vi "Read Excel data.vi"() -> (0 "Number of rows":i32, 1 "Plot Group":dbl[][](array[numeric]), 2 "Voltage Offsets":dbl[][](array[numeric]), 3 "Chirp Durations":dbl[][](array[numeric]))   [LabVIEW 2017]
uses:
  <vilib>/Utility/file.llb/Read Delimited Spreadsheet (DBL).vi
panel:
  out "array w/o headers":dbl[][](array[numeric])
  out "all rows":dbl[][](array[numeric])
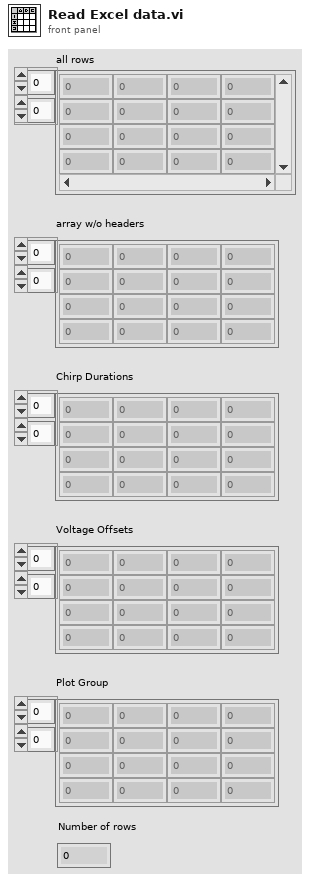
[diagram p1: front panel]
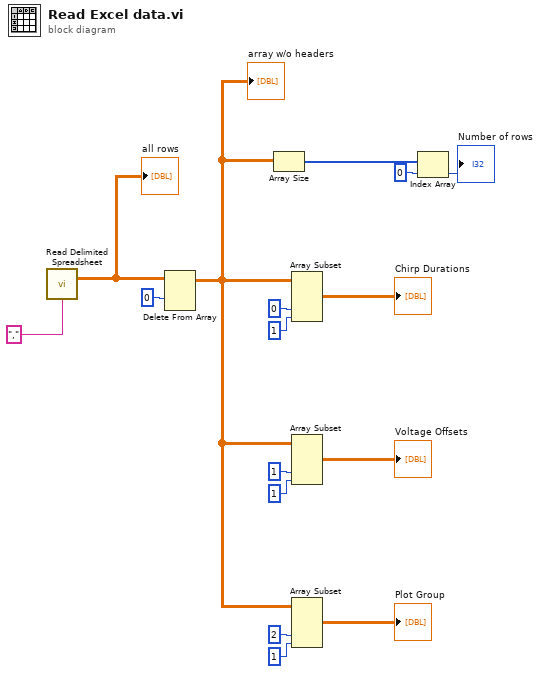
[diagram p0: block diagram]
diagram:
  n1 = call-poly <vilib>:"Read Delimited Spreadsheet.vi"("delimiter (\\t)"="," ("delimiter (\\t)")) -> ("all rows"=w16:dbl[][])  [unwired: 9 in, 5 out]
  "all rows" <- w16
  n2 = Delete From Array(array=w16, index (row)=0) -> (array with subset deleted=w4:dbl[][])  [unwired: 2 in, 1 out]
  "array w/o headers" <- w4
  n3 = Array Size(array=w4) -> (size(s)=w3:i32[])
  n4 = Array Subset(array=w4, index (col)=0 ("index"), length (col)=1 ("length")) -> (→"Chirp Durations":dbl[][])  [unwired: 2 in]
  n5 = Array Subset(array=w4, index (col)=1 ("index"), length (col)=1 ("length")) -> (→"Voltage Offsets":dbl[][])  [unwired: 2 in]
  n6 = Array Subset(array=w4, index (col)=2 ("index"), length (col)=1 ("length")) -> (→"Plot Group":dbl[][])  [unwired: 2 in]
  n7 = Index Array(array=w3, index=0) -> (element=→"Number of rows":i32)
